vi "Set Material.vi"(4 "Diffuse":T2, 5 "Specular":T2, 6 "Emission":T2, 7 "Ambient":T2, 8 "error in (no error)":errorcluster, 9 "Shininess":sgl, 10 "Color Mode":T1(ring), 11 "Scene Object In":refnum<vi>) -> (0 "error out":errorcluster, 3 "Scene Object Out":refnum<vi>)   [LabVIEW 2017, in "NI_3D Picture Control.lvlib"]
doc: "Specifies surface properties used by lighting equations during rendering. Inputs specified by this VI appear only in lit scenes."
uses:
  <vilib>/picture/3D Picture Control/NI_3D Picture Control.lvlib
  <vilib>/Utility/miscctls.llb/LVRGBAColorTypeDef.ctl
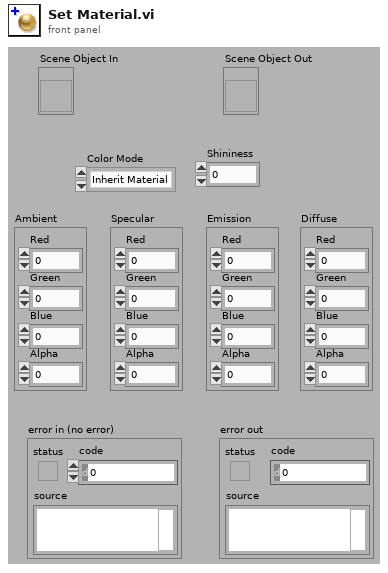
[diagram p1: front panel]
types:
  T1 = enum16{"Inherit Material", "Use entire Material", "Ignore Ambient", "Ignore Diffuse", "Ignore Specular", "Ignore Emission", "Ignore Ambient and Diffuse"}
  T2 = typedef "LVRGBAColorTypeDef.ctl" = cluster{"Red":sgl, "Green":sgl, "Blue":sgl, "Alpha":sgl}
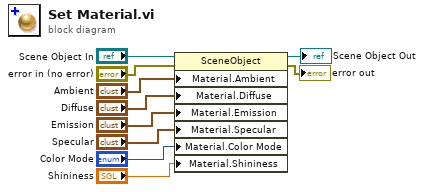
[diagram p0: block diagram]
diagram:
  n1 = property class="SceneObject"(reference="Scene Object In", error in="error in (no error)", "Material.Ambient"="Ambient", "Material.Diffuse"="Diffuse", "Material.Emission"="Emission", "Material.Specular"="Specular", "Material.Color Mode"="Color Mode", "Material.Shininess"="Shininess") -> (reference out=→"Scene Object Out":refnum<vi>, error out=→"error out":errorcluster)
